vi "Configure Temperature (RTD).vi"(0 "VISA resource name":refnum<visa-resource-name>, 1 "Unit (1: Celsius)":i32(ring)=1 items=["Kelvin", "Celsius", "Fahrenheit"], 2 "Delta (1.4999)":dbl=1.4999, 3 "Alpha (0.00385055)":dbl=0.00385055, 7 "RTD Type (0: PT100)":i32(ring) items=["PT100", "PT385", "PT3916", "D100", "F100", "USER"], 9 "Channel List(\"\")":string, 11 "error in (no error)":errorcluster, 12 "Wire Number (0: Four)":i32(ring) items=["Four", "Three", "Two"], 13 "Beta (0.10863)":dbl=0.10863, 14 "Zero (100)":dbl=100.0) -> (4 "VISA resource name out":refnum<visa-resource-name>, 15 "error out":errorcluster)   [LabVIEW 2019, in "Keithley DMM6500 DAQ6500 Series.lvlib"]
doc: "Configures the temperature thremal sensor with RTD."
uses:
  Keithley DMM6500 DAQ6500 Series.lvlib
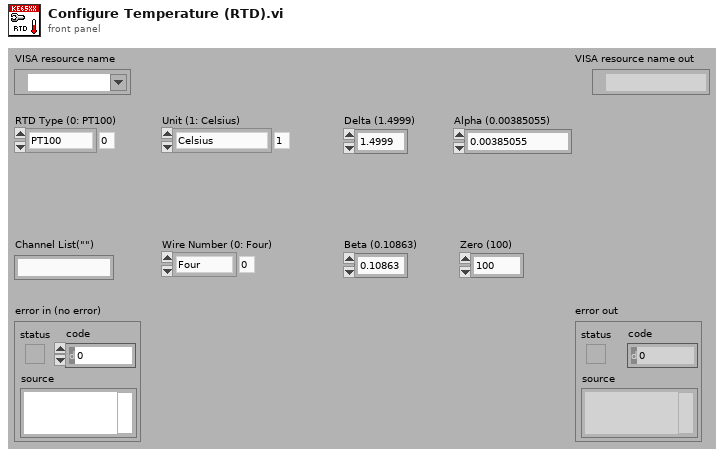
[diagram p1: front panel]
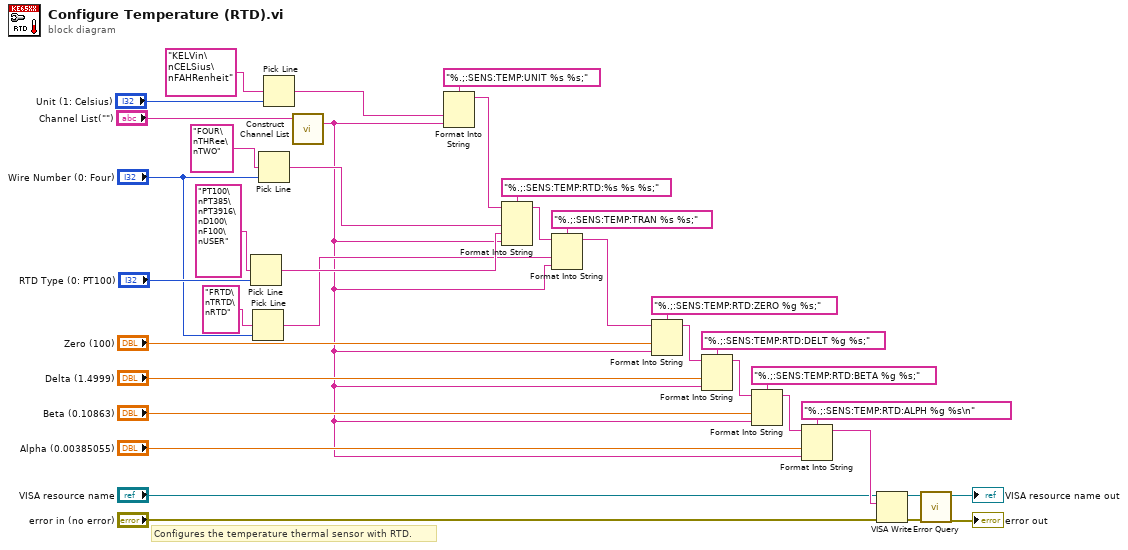
[diagram p0: block diagram]
diagram:
  # "Configures the temperature thermal sensor with RTD."
  n1 = Pick Line(multi-line string="PT100\nPT385\nPT3916\nD100\nF100\nUSER", line index="RTD Type (0: PT100)") -> (output string=w11:string)  [unwired: 1 in]
  n2 = Pick Line(multi-line string="FRTD\nTRTD\nRTD", line index="Wire Number (0: Four)") -> (output string=w6:string)  [unwired: 1 in]
  n3 = Pick Line(multi-line string="FOUR\nTHRee\nTWO", line index="Wire Number (0: Four)") -> (output string=w14:string)  [unwired: 1 in]
  n4 = Pick Line(multi-line string="KELVin\nCELSius\nFAHRenheit", line index="Unit (1: Celsius)") -> (output string=w10:string)  [unwired: 1 in]
  n5 = call "Construct Channel List.vi"("Channel List"="Channel List(\"\")") -> ("Channel List String"=w1:string)  [unwired: 2 in]
  n6 = Format Into String(format string="%.;:SENS:TEMP:UNIT %s %s;", w10, w1) -> (resulting string=w16:string)  [unwired: 2 in, 1 out]
  n7 = Format Into String(format string="%.;:SENS:TEMP:RTD:%s %s %s;", initial string=w16, w14, w11, w1) -> (resulting string=w36:string)  [unwired: 1 in, 1 out]
  n8 = Format Into String(format string="%.;:SENS:TEMP:TRAN %s %s;", initial string=w36, w6, w1) -> (resulting string=w9:string)  [unwired: 1 in, 1 out]
  n9 = Format Into String(format string="%.;:SENS:TEMP:RTD:ZERO %g %s;", initial string=w9, "Zero (100)", w1) -> (resulting string=w33:string)  [unwired: 1 in, 1 out]
  n10 = Format Into String(format string="%.;:SENS:TEMP:RTD:DELT %g %s;", initial string=w33, "Delta (1.4999)", w1) -> (resulting string=w31:string)  [unwired: 1 in, 1 out]
  n11 = Format Into String(format string="%.;:SENS:TEMP:RTD:BETA %g %s;", initial string=w31, "Beta (0.10863)", w1) -> (resulting string=w29:string)  [unwired: 1 in, 1 out]
  n12 = Format Into String(format string="%.;:SENS:TEMP:RTD:ALPH %g %s\n", initial string=w29, "Alpha (0.00385055)", w1) -> (resulting string=w27:string)  [unwired: 1 in, 1 out]
  n13 = VISA Write(VISA resource name="VISA resource name", write buffer=w27, error in (no error)="error in (no error)") -> (VISA resource name out=w24:refnum<visa-resource-name>, error out=w23:errorcluster)  [unwired: 1 out]
  n14 = call "Error Query.vi"("error in (no error)"=w23, "VISA resource name"=w24) -> ("error out"=→"error out":errorcluster, "VISA resource name out"=→"VISA resource name out":refnum<visa-resource-name>)  [unwired: 6 in, 2 out]
